vi "PlayWave_multchannel.vi"() -> ()   [LabVIEW 2016]
uses:
  <vilib>/measure/NI_MABase.lvlib
panel:
  in  "Direction (Record)":u16(ring)=1 items=["Record", "Play", "Loopback", "ASIO input", "ASIO output", "Record (WASAPI)", "Play (WASAPI)"]
  in  "device (0)":u32
  in  "Frequencies":dbl[](array[numeric])=[100.0, 300.0, 500.0, 700.0, 900.0, 1100.0]
  out "Device Names":string[](array[string])
  out "Number of Output Devices":i32=2
  out "Play Error":errorcluster
  in  "Format":cluster{"Rate":i32, "Bits":i32, "Channels":i32}={"Rate"=44100, "Bits"=16, "Channels"=2}
  in  "Buffer":T1={"# buffers"=4, "Buffer size"=2000, "unit (ms)"=enum."Samples"}
  out "error out":errorcluster={"status"=TRUE, "code"=-20, "source"="WaveIO: Input Data do not match Format"}
  out "Waveform Graph":i32[][](graph)
  in  "Stop":bool
  # "Play multiple channels (up to 6) on sound card"
  # "JUST FOR INFORMATION\nHas no effect in the code!!"
  # "Greater than 1000"
  # "DO NOT CHANGE"
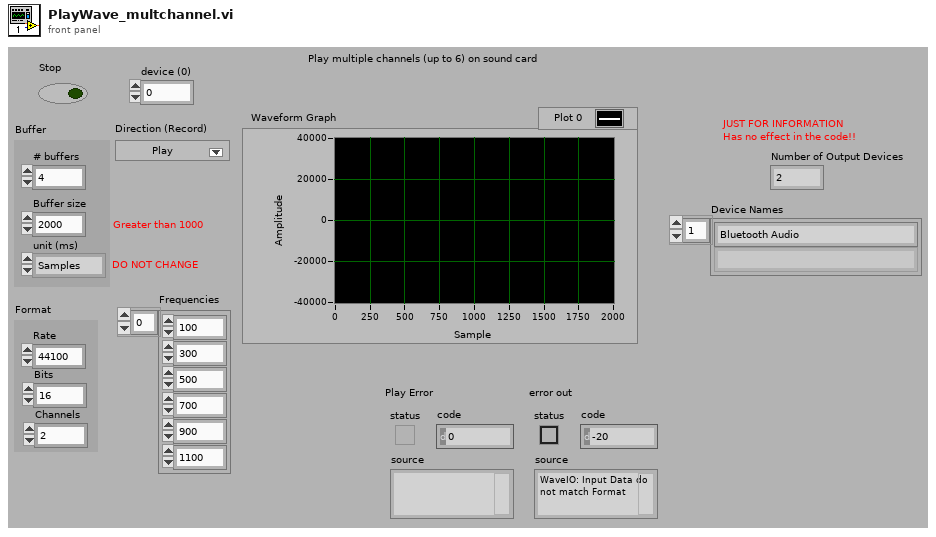
[diagram p1: front panel]
types:
  T1 = cluster{"# buffers":i32, "Buffer size":i32, "unit (ms)":enum16{"time (ms)", "Samples"}}
  T2 = enum16{"Sine Wave", "Triangle Wave", "Square Wave", "Sawtooth Wave"}
  T3 = typedef "SoundHandle.ctl" = cluster{"DeviceID":u16, "Samples/buf":u32, "Sampl rate":u32, "Bits/sample":u16, "Channels":u8, "Opened":bool}
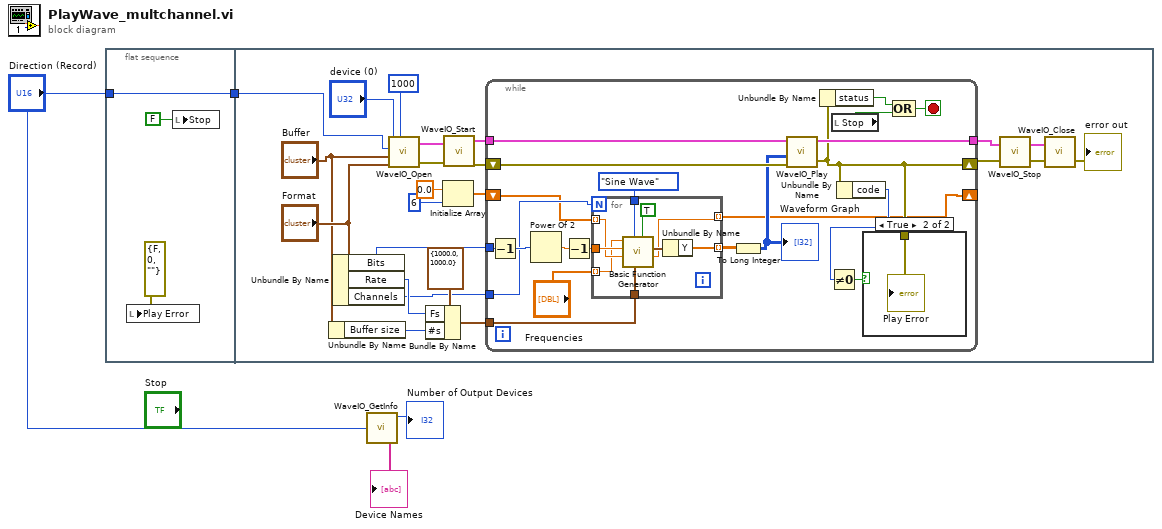
[diagram p0: block diagram]
diagram:
  n1 = flat-sequence {
    tunnel: [w5] -> w2
    tunnel: "Direction (Record)" -> [w5]
    tunnel: w2 -> [w8]
    frame #0 {
      n2 = local write "Play Error"(errorcluster {"status"=FALSE, "code"=0, "source"=""} ("Play Error")) -> ()
      n3 = local write "Stop"(FALSE ("Stop")) -> ()
    }
    frame #1 {
      n4 = Unbundle By Name("Buffer") -> ("Buffer size"=w15:i32)
      n5 = Unbundle By Name("Format") -> ("Bits"=w14:i32, "Rate"=w17:i32, "Channels"=w10:i32)
      n6 = call "WaveIO_Open.vi"("idev"="device (0)", "Watchdog timeout (msec) (default=OFF)"=1000, "device type (Record)"=w8, "Buffer Config"="Buffer", "Format (44kHz, 16Bit, stereo)"="Format") -> ("Sound Handle Out"=w22:T3, "error out"=w21:errorcluster)  [unwired: 2 in]
      n7 = Bundle By Name(cluster=cluster{"Fs":dbl, "#s":dbl} {"Fs"=1000.0, "#s"=1000.0} ("sampling info"), "Fs"=w17, "#s"=w15) -> (w25:cluster{"Fs":dbl, "#s":dbl})
      n8 = Initialize Array(0.0 ("element"), 6 ("dimension size")) -> (w13:dbl[])
      n9 = call "WaveIO_Start.vi"("error in (no error)"=w21, "Handle"=w22) -> ("error out"=w23:errorcluster, "Handle Out"=w24:T3)
      n10 = while {
        shift-right: [w37] -> w20
        shift-left: w23 -> [w48]
        tunnel: w24 -> [w49]
        tunnel: [w45] -> w29
        tunnel: w25 -> [w46]
        tunnel: w14 -> [w43]
        shift-right: [w32] -> _
        shift-left: w13 -> [w33]
        tunnel: w10 -> [w34]
        stop <- w51 stop-if-true
        n11 = Decrement(x=w43) -> (x-1=w41:i32)
        n12 = Power Of 2(x=w41) -> (2^x=w42:dbl)
        n13 = Decrement(x=w42) -> (x-1=w40:dbl)
        n14 = for {
          N: w34 -> [_]
          tunnel: w46 -> [w59]
          tunnel: T2."Sine Wave" ("signal type") -> [w58]
          tunnel: w40 -> [w57]
          tunnel: [w56] -> w36 mode=indexing
          tunnel: w33 -> [w55] mode=indexing
          tunnel: [w54] -> w32 mode=indexing
          tunnel: "Frequencies" -> [w52] mode=indexing
          n15 = call <vilib>:"Basic Function Generator.vi"("reset signal"=TRUE, "sampling info"=w59, "signal type"=w58, "phase"=w55, "amplitude"=w57, "frequency"=w52) -> ("phase out"=w54:dbl, "signal out"=w60:waveform(dbl))  [unwired: 3 in, 1 out]
          n16 = Unbundle By Name(w60) -> ("Y"=w56:dbl[])
        }
        n17 = To Long Integer(number=w36) -> (32bit integer=w35:i32[][])
        "Waveform Graph" <- w35
        n18 = call "WaveIO_Play.vi"("error in (no error)"=w48, "data"=w35, "Handle"=w49) -> ("error out"=w37:errorcluster, "Handle Out"=w45:T3)  [unwired: 1 in]
        n19 = Unbundle By Name(w37) -> ("status"=w50:bool)
        n20 = local read "Stop"() -> (w47:bool)
        n21 = Unbundle By Name(w37) -> ("code"=w38:i32)
        n22 = Not Equal To 0?(x=w38) -> (x != 0?=w39:bool)
        n23 = case shown="True" w39 {
          tunnel: w37 -> [_ w61]
          frame False {
          }
          frame True {
            "Play Error" <- w61
          }
        }
        n24 = Compound Arithmetic op=OR(w50, w47) -> (w51:bool)
      }
      n25 = call "WaveIO_Stop.vi"("error in (no error)"=w20, "Handle"=w29) -> ("error out"=w27:errorcluster, "Handle Out"=w30:T3)
      n26 = call "WaveIO_Close.vi"("error in (no error)"=w27, "Handle"=w30) -> ("error out"=→"error out":errorcluster)  [unwired: 1 out]
    }
  }
  n27 = call "WaveIO_GetInfo.vi"("Direction (Input)"="Direction (Record)") -> ("numdev"=→"Number of Output Devices":i32, "Dev Names"=→"Device Names":string[])  [unwired: 2 out]
